vi "smart_home (1).vi"() -> ()   [LabVIEW 2017]
uses:
  <vilib>/MakerHub/LINX/Public/Peripherals/Analog/Analog Read 1 Chan.vi
  <vilib>/MakerHub/LINX/Public/Peripherals/Digital/Digital Write 1 Chan.vi
  <vilib>/MakerHub/LINX/Public/Peripherals/Digital/Digital Read 1 Chan.vi
  <vilib>/MakerHub/LINX/Public/Peripherals/Analog/Analog Read N Chans.vi
  <vilib>/MakerHub/LINX/Public/Peripherals/Digital/Digital Write N Chans.vi
  <vilib>/MakerHub/LINX/Public/Peripherals/Digital/Digital Read N Chans.vi
  <vilib>/MakerHub/LINX/Private/Local IO/LinxAnalogRead.vi
  <vilib>/MakerHub/LINX/Public/Utilities/Check Channel.vi
  <vilib>/MakerHub/LINX/Private/Local IO/LinxDigitalWrite.vi
  <vilib>/MakerHub/LINX/Private/Local IO/LinxDigitalRead.vi
  <vilib>/MakerHub/LINX/Public/Utilities/Open Serial.vi
  <vilib>/MakerHub/LINX/Public/Sensors/Motion/Servo/Servo Open One Channel.vi
  <vilib>/MakerHub/LINX/Public/Sensors/Motion/Servo/Servo Set Pulse Width One Channel.vi
  <vilib>/MakerHub/LINX/Private/Utilties/Generate Error.vi
  <vilib>/MakerHub/LINX/Public/Sensors/Motion/Servo/Servo Close One Channel.vi
  <vilib>/MakerHub/LINX/LMH-LINX.lvlib
  <vilib>/MakerHub/LINX/Public/Sensors/Motion/Servo/Servo.lvlib
panel:
  out "W 5":bool
  out "W 4":bool
  out "W 3":bool
  out "W 2":bool
  out "W 1":bool
  out "Rs/Ro(MQ2)":dbl
  out "Rs(MQ2)":dbl
  out "Boolean":bool
  out "Smoke  Graph":dbl[](graph)
  out "Smoke PPM2":dbl[](array[numeric])
  out "Smoke":dbl(knob) scale=0.0..10000.0
  out "alarm 2":bool
  in  "Servo Channel":u8
  in  "Dial":dbl(knob) scale=500.0..2500.0
  out "Waveform Chart 2":dbl(graph)
  out "Thermometer 2":dbl(slide) scale=0.0..60.0
  in  "Serial Port 2":refnum<visa-resource-name>="N/A"
  in  "Stop Button 2":bool
  in  "LED Value":bool
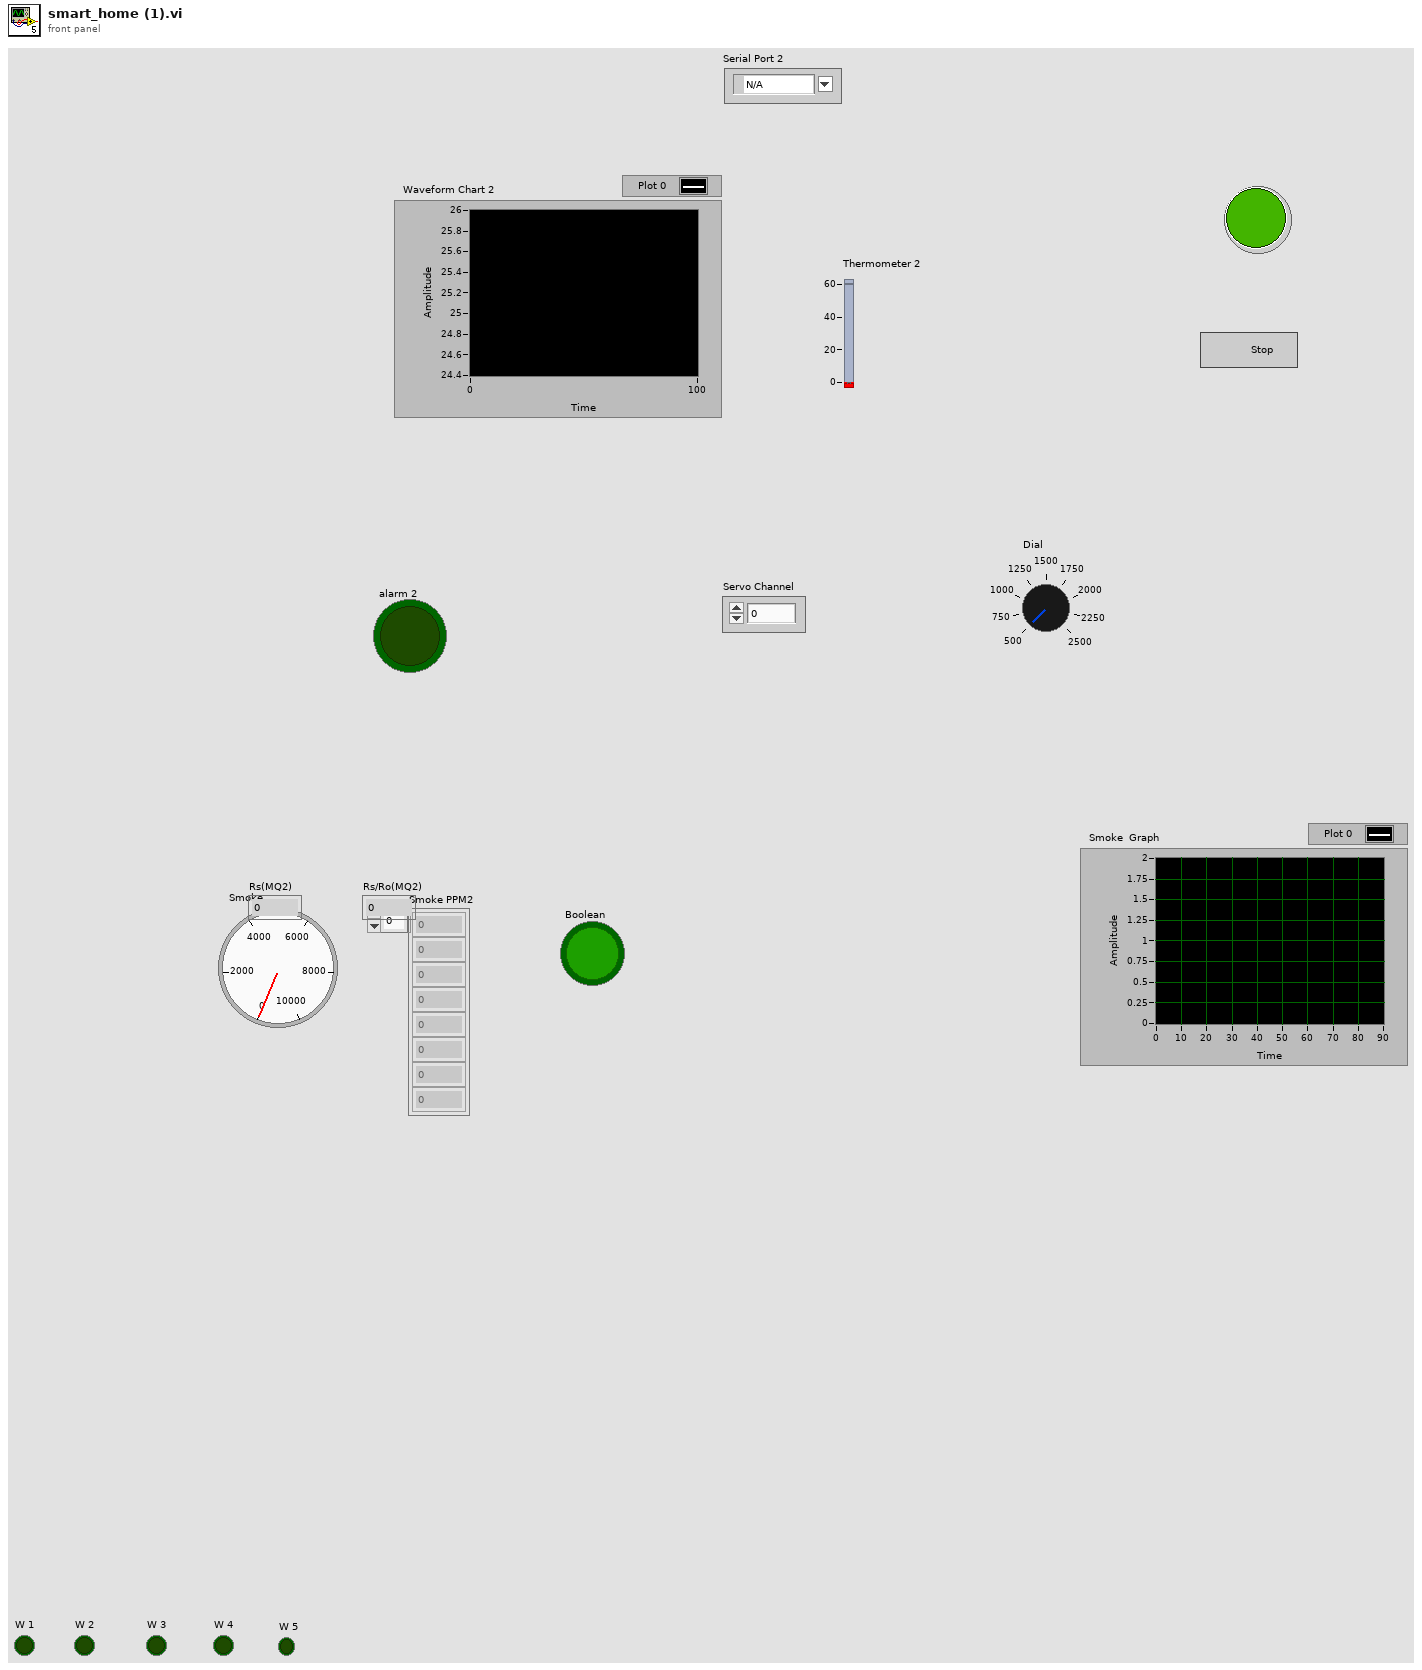
[diagram p1: front panel]
types:
  T1 = typedef "LMH-LINX.lvlib/LINX Ref.ctl" = cluster{"IO":T2, "Interface":T3, "LINX Device Config":T4}
  T2 = typedef "LMH-LINX.lvlib/Platform.ctl" = enum16{"Remote", "Local"}
  T3 = typedef "LMH-LINX.lvlib/Interface.ctl" = enum16{"Serial", "TCP"}
  T4 = typedef "LMH-LINX.lvlib/Device.lvlib/LINX Device Config.ctl" = cluster{"Interface":T3, "COM Port":refnum<visa-resource-name>, "TCP Configuration":T5, "Device Family":u8, "Device ID":u8, "Device Name":string, "TCP Ref":refnum<k5>, "Channels":T6}
  T5 = typedef "LMH-LINX.lvlib/Device.lvlib/TCP Config.ctl" = cluster{"IP Address":string, "Port":u16}
  T6 = typedef "LMH-LINX.lvlib/Channels.ctl" = cluster{"DI":u8[], "DO":u8[], "AI":u8[], "AO":u8[], "PWM":u8[], "QE":u8[], "UART":u8[], "I2C 2":u8[], "SPI":u8[], "CAN":u8[], "Servo":u8[], "AI Ref (V)":dbl, "AI Resolution (Bits)":u8, "AO Ref (V)":dbl, "AO Resolution (Bits)":u8}
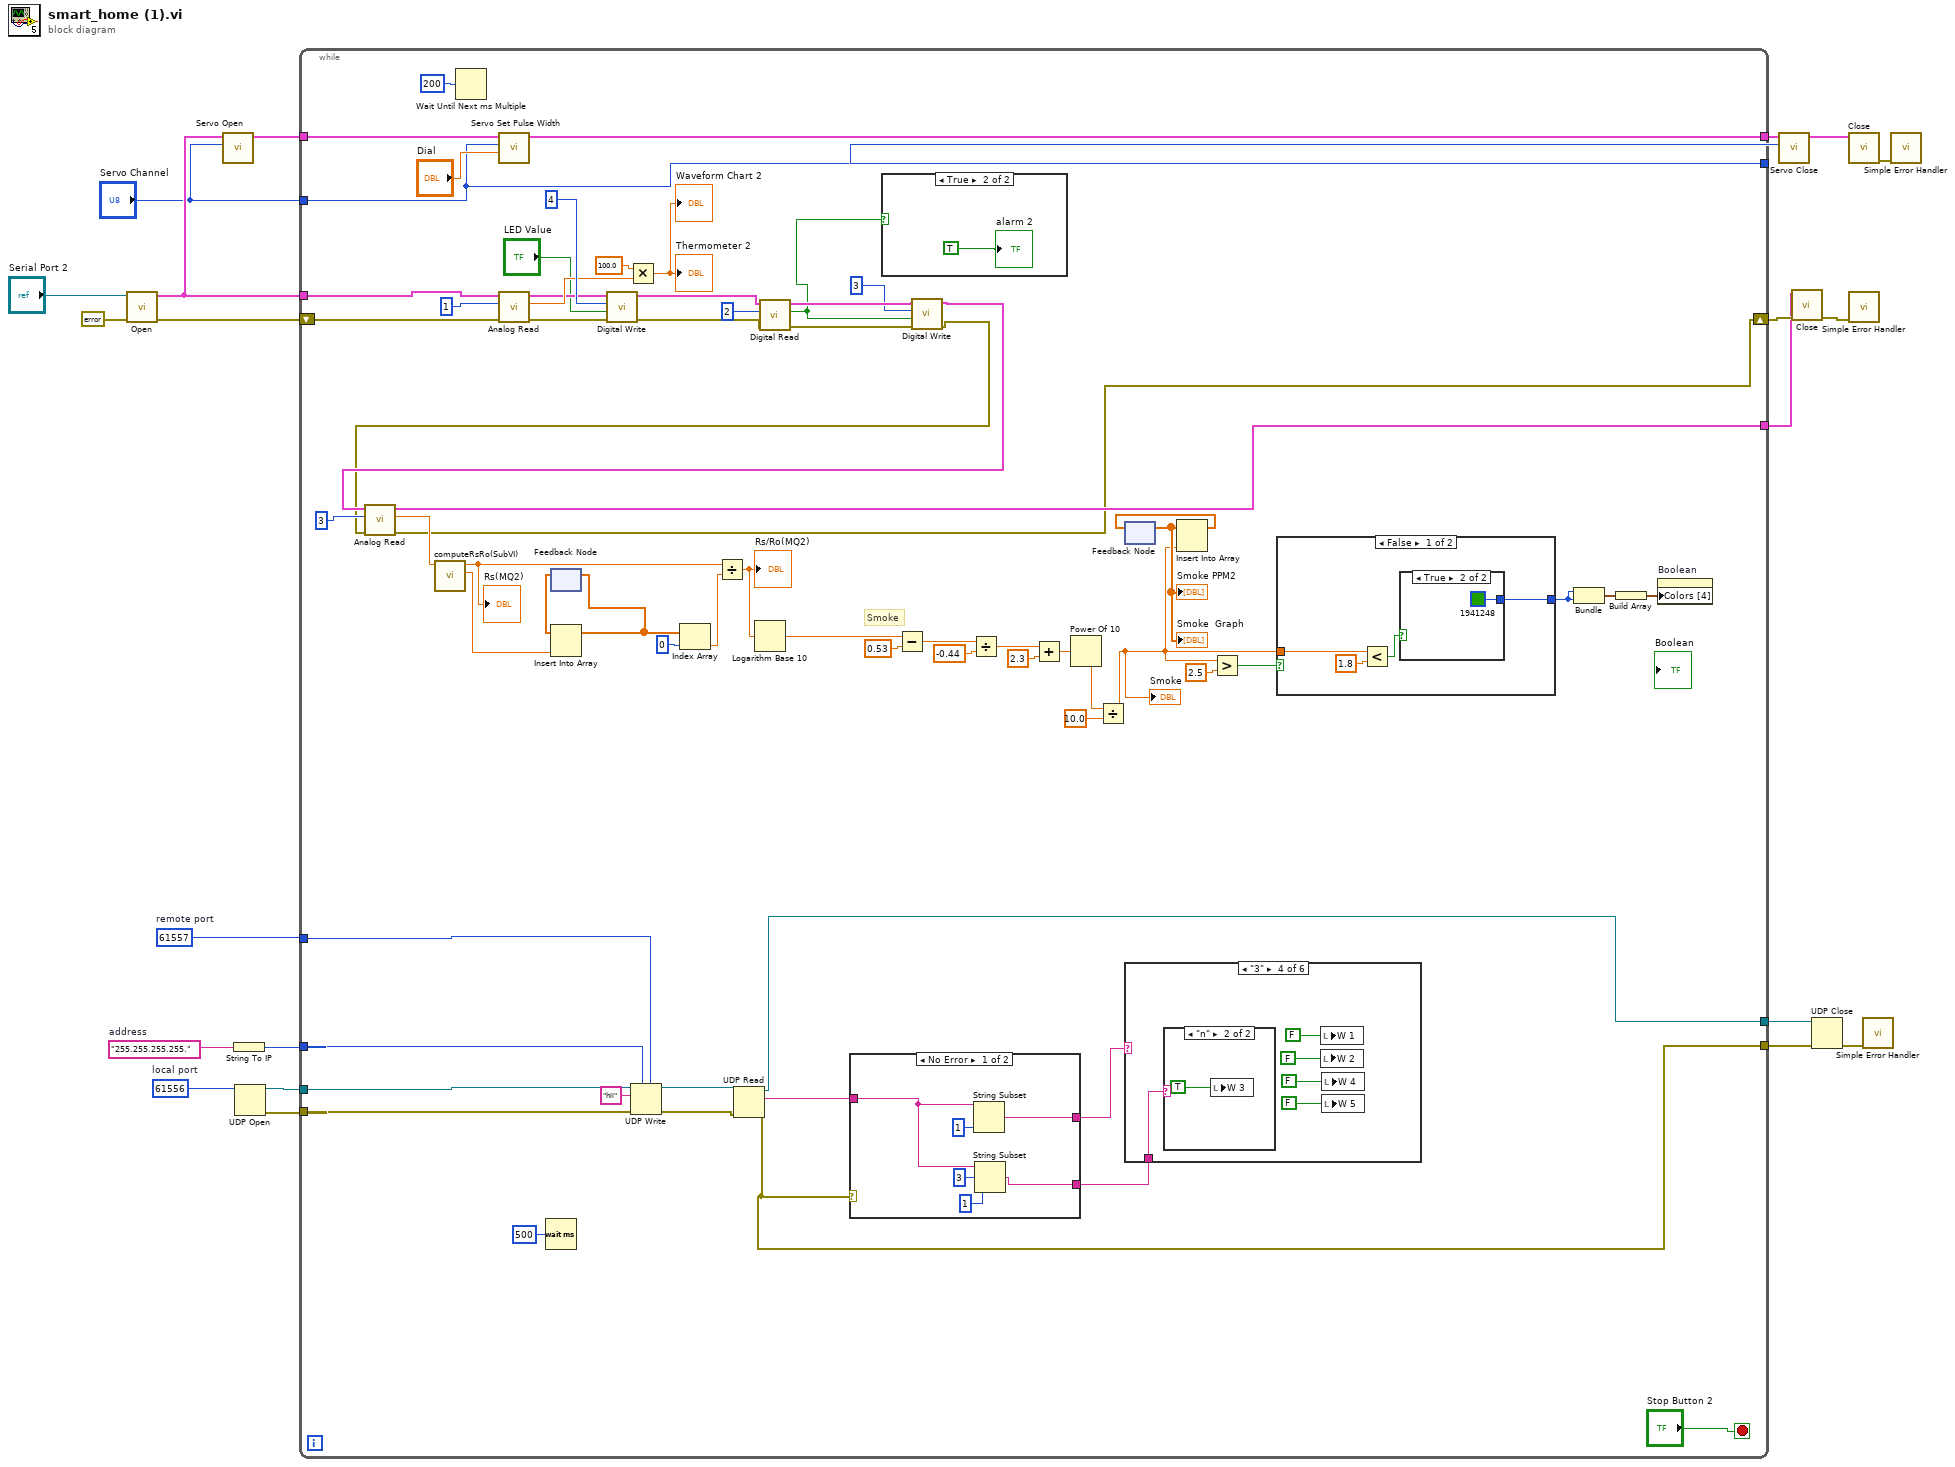
[diagram p0: block diagram]
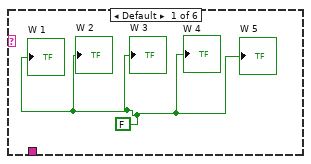
[diagram p2: hidden frame]
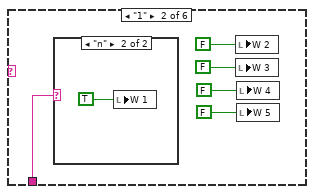
[diagram p3: hidden frame]
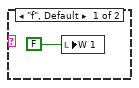
[diagram p4: hidden frame]
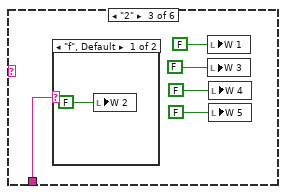
[diagram p5: hidden frame]
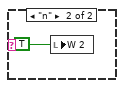
[diagram p6: hidden frame]
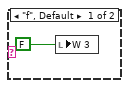
[diagram p7: hidden frame]
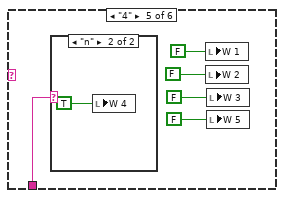
[diagram p8: hidden frame]
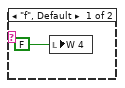
[diagram p9: hidden frame]
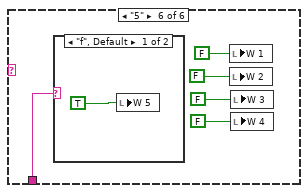
[diagram p10: hidden frame]
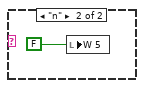
[diagram p11: hidden frame]
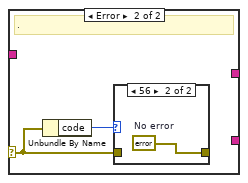
[diagram p12: hidden frame]
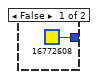
[diagram p14: hidden frame]
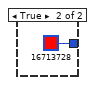
[diagram p15: hidden frame]
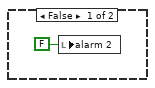
[diagram p16: hidden frame]
diagram:
  w7 = u16 61557  # remote port
  w8 = u16 61556  # local port
  w9 = "255.255.255.255."  # address
  n1 = call-poly <vilib>:"Open.vi"("Error In"=errorcluster {"status"=FALSE, "code"=0, "source"=""}, "Serial Port"="Serial Port 2") -> ("Error Out"=w22:errorcluster, "LINX Resource"=w18:T1)  [unwired: 7 in, 1 out]
  n2 = call-poly <vilib>:"Servo Open.vi"("Servo Channel"="Servo Channel", "LINX Resource"=w18) -> ("LINX Resource"=w17:T1)  [unwired: 8 in, 1 out]
  n3 = String To IP(1:w9) -> (0:w6:u32)
  n4 = UDP Open(11:w8) -> (port=w5:refnum<k16>, 0:w4:errorcluster)  [unwired: 4 in, 1 out]
  n5 = while {
    tunnel: w18 -> [w82]
    shift-right: [w39] -> w21
    shift-left: w22 -> [w80]
    tunnel: w17 -> [w76]
    tunnel: [w75] -> w16
    tunnel: "Servo Channel" -> [w74]
    tunnel: [w74] -> w14
    tunnel: [w41] -> w11
    tunnel: w7 -> [w28]
    tunnel: w6 -> [w27]
    tunnel: w5 -> [w26]
    tunnel: w4 -> [w25]
    tunnel: [w24] -> w2
    tunnel: [w23] -> w1
    stop <- "Stop Button 2" stop-if-true
    # "Smoke"
    n6 = Wait Until Next ms Multiple(millisecond multiple=u32 200) -> ()  [unwired: 1 out]
    n7 = call-poly <vilib>:"Servo Set Pulse Width.vi"("Pulse Width (uS)"="Dial", "Servo Channel"=w74, "LINX Resource"=w76) -> ("LINX Resource"=w75:T1)  [unwired: 7 in, 1 out]
    n8 = call-poly <vilib>:"Analog Read.vi"("Error In"=w80, "Analog Channel"=u8 1 ("DI Channel"), "LINX Resource"=w82) -> ("Error Out"=w79:errorcluster, "Voltage"=w84:dbl, "LINX Resource"=w81:T1)  [unwired: 5 in, 1 out]
    n9 = Wait (ms)(milliseconds to wait=u32 500) -> ()  [unwired: 1 out]
    n10 = feedback #1() -> (w47:dbl[])  [unwired: 1 in]
    n11 = call-poly <vilib>:"Digital Write.vi"("Error In"=w79, "Output Value"="LED Value", "DO Channel"=u8 4 ("Digital Output Channel"), "LINX Resource"=w81) -> ("Error Out"=w72:errorcluster, "LINX Resource"=w73:T1)  [unwired: 6 in]
    n12 = Multiply(x=100.0, y=w84) -> (x*y=→"Thermometer 2" →"Waveform Chart 2":dbl)
    n13 = UDP Write(address=w27, port or service name=w28, connection ID=w26, data in="hii", 8:w25) -> (error out=w32:errorcluster, 3:w33:refnum<k16>)  [unwired: 1 in]
    n14 = UDP Read(connection ID=w33, 8:w32) -> (data out=w29:string, error out=w23:errorcluster, 3:w24:refnum<k16>)  [unwired: 2 in, 2 out]
    n15 = call-poly <vilib>:"Digital Read.vi"("Error In"=w72, "DI Channel"=u8 2, "LINX Resource"=w73) -> ("Error Out"=w69:errorcluster, "DI Value"=w68:bool, "LINX Resource"=w70:T1)  [unwired: 6 in]
    n16 = case shown="No Error" w23 {
      selector: w23 -> [_ w131]
      tunnel: [w127 _] -> w31
      tunnel: [w126 _] -> w30
      tunnel: w29 -> [w125 _]
      frame No Error {
        n17 = String Subset(string=w125, length (rest)=1 ("length (rest)")) -> (substring=w127:string)  [unwired: 1 in]
        n18 = String Subset(string=w125, offset (0)=3, length (rest)=1 ("length (rest)")) -> (substring=w126:string)
      }
      frame Error {
        # "."
        n19 = Unbundle By Name(w131) -> ("code"=w132:i32)
        n20 = case shown="56" w132 {
          tunnel: w131 -> [w133 _]
          tunnel: [w133 w134] -> _
          frame Default {
          }
          frame 56 {
            w134 = errorcluster {"status"=FALSE, "code"=0, "source"=""}  # No error
          }
        }
      }
    }
    n21 = case shown="True" w68 {
      frame False {
        n22 = local write "alarm 2"(FALSE ("alarm 2")) -> ()
      }
      frame True {
        "alarm 2" <- TRUE ("alarm")
      }
    }
    n23 = call-poly <vilib>:"Digital Write.vi"("Error In"=w69, "Output Value"=w68, "DO Channel"=u8 3, "LINX Resource"=w70) -> ("Error Out"=w40:errorcluster, "LINX Resource"=w42:T1)  [unwired: 6 in]
    n24 = call-poly <vilib>:"Analog Read.vi"("Error In"=w40, "Analog Channel"=u8 3, "LINX Resource"=w42) -> ("Error Out"=w39:errorcluster, "Voltage"=w57:dbl, "LINX Resource"=w41:T1)  [unwired: 5 in, 1 out]
    n25 = call "computeRsRo(SubVI).vi"("Voltage"=w57) -> ("Ro"=w48:dbl, "Rs"=w44:dbl)  [unwired: 9 in]
    "Rs(MQ2)" <- w44
    n26 = Insert Into Array "Insert Into Array"(array=w47, new element=w48) -> (w46:dbl[])  [unwired: 1 in]
    n27 = feedback-in #1(w46) -> ()
    n28 = Index Array(array=w46, index=0) -> (element=w45:dbl)
    n29 = Divide(x=w44, y=w45) -> (x/y=w56:dbl)
    "Rs/Ro(MQ2)" <- w56
    n30 = Logarithm Base 10(1:w56) -> (0:w55:dbl)
    n31 = Subtract(x=w55, y=0.53) -> (x-y=w53:dbl)
    n32 = Divide(x=w53, y=-0.44) -> (x/y=w51:dbl)
    n33 = Add(x=w51, y=2.3) -> (x+y=w65:dbl)
    n34 = Power Of 10(x=w65) -> (10^x=w37:dbl)
    n35 = Divide(x=w37, y=10.0) -> (x/y=w38:dbl)
    "Smoke" <- w38
    n36 = feedback #2() -> (w58:dbl[])  [unwired: 1 in]
    "Smoke PPM2" <- w58
    "Smoke  Graph" <- w58
    n37 = case shown="\"3\"" w31 {
      tunnel: w30 -> [_ w90 w97 w104 w111 w118]
      frame Default {
        w89 = FALSE
        "W 5" <- w89
        "W 4" <- w89
        "W 3" <- w89
        "W 2" <- w89
        "W 1" <- w89
      }
      frame "1" {
        n38 = case shown="\"n\"" w90 {
          frame "f", Default {
            n39 = local write "W 1"(FALSE ("Boolean")) -> ()
          }
          frame "n" {
            n40 = local write "W 1"(TRUE ("Boolean")) -> ()
          }
        }
        n41 = local write "W 2"(FALSE ("Boolean 2")) -> ()
        n42 = local write "W 3"(FALSE ("Boolean 3")) -> ()
        n43 = local write "W 4"(FALSE ("Boolean 4")) -> ()
        n44 = local write "W 5"(FALSE ("Boolean 5")) -> ()
      }
      frame "2" {
        n45 = case shown="\"f\", Default" w97 {
          frame "f", Default {
            n46 = local write "W 2"(FALSE ("Boolean 2")) -> ()
          }
          frame "n" {
            n47 = local write "W 2"(TRUE ("Boolean 2")) -> ()
          }
        }
        n48 = local write "W 1"(FALSE ("Boolean")) -> ()
        n49 = local write "W 3"(FALSE ("Boolean 3")) -> ()
        n50 = local write "W 4"(FALSE ("Boolean 4")) -> ()
        n51 = local write "W 5"(FALSE ("Boolean 5")) -> ()
      }
      frame "3" {
        n52 = case shown="\"n\"" w104 {
          frame "f", Default {
            n53 = local write "W 3"(FALSE ("Boolean 3")) -> ()
          }
          frame "n" {
            n54 = local write "W 3"(TRUE ("Boolean 3")) -> ()
          }
        }
        n55 = local write "W 1"(FALSE ("Boolean")) -> ()
        n56 = local write "W 2"(FALSE ("Boolean 2")) -> ()
        n57 = local write "W 4"(FALSE ("Boolean 4")) -> ()
        n58 = local write "W 5"(FALSE ("Boolean 5")) -> ()
      }
      frame "4" {
        n59 = case shown="\"n\"" w111 {
          frame "f", Default {
            n60 = local write "W 4"(FALSE ("Boolean 4")) -> ()
          }
          frame "n" {
            n61 = local write "W 4"(TRUE ("Boolean 4")) -> ()
          }
        }
        n62 = local write "W 1"(FALSE ("Boolean")) -> ()
        n63 = local write "W 2"(FALSE ("Boolean 2")) -> ()
        n64 = local write "W 3"(FALSE ("Boolean 3")) -> ()
        n65 = local write "W 5"(FALSE ("Boolean 5")) -> ()
      }
      frame "5" {
        n66 = case shown="\"f\", Default" w118 {
          frame "f", Default {
            n67 = local write "W 5"(TRUE ("Boolean 6")) -> ()
          }
          frame "n" {
            n68 = local write "W 5"(FALSE ("Boolean 5")) -> ()
          }
        }
        n69 = local write "W 1"(FALSE ("Boolean")) -> ()
        n70 = local write "W 2"(FALSE ("Boolean 2")) -> ()
        n71 = local write "W 3"(FALSE ("Boolean 3")) -> ()
        n72 = local write "W 4"(FALSE ("Boolean 4")) -> ()
      }
    }
    n73 = Insert Into Array(array=w58, new element=w38) -> (w64:dbl[])  [unwired: 1 in]
    n74 = feedback-in #2(w64) -> ()
    n75 = Greater?(x=w38, y=2.5) -> (0:w63:bool)
    n76 = case shown="False" w63 {
      tunnel: [w136 u32 16713728] -> w61
      tunnel: w38 -> [w135 _]
      frame False {
        n77 = Less?(x=w135, y=1.8) -> (x < y?=w138:bool)
        n78 = case shown="True" w138 {
          tunnel: [u32 16772608 u32 1941248] -> w136
          frame False {
          }
          frame True {
          }
        }
      }
      frame True {
      }
    }
    n79 = Bundle(w61, w61) -> (w60:cluster{u32, u32})  [unwired: 1 in]
    n80 = Build Array(w60) -> (w59:cluster{u32, u32}[])
    n81 = property on="Boolean" class="Bool (strict)"("Colors [4]"=w59) -> ()  [unwired: 2 in, 2 out]
  }
  n82 = call-poly <vilib>:"Servo Close.vi"("Servo Channel"=w14, "LINX Resource"=w16) -> ("LINX Resource"=w12:T1)  [unwired: 8 in, 1 out]
  n83 = call <vilib>:"Close.vi"("Error In"=w21, "LINX Resource"=w11) -> ("Error Out"=w20:errorcluster)  [unwired: 9 in]
  n84 = UDP Close(connection ID=w2, 8:w1) -> (error out=w3:errorcluster)  [unwired: 1 out]
  n85 = call <vilib>:"Close.vi"("LINX Resource"=w12) -> ("Error Out"=w13:errorcluster)  [unwired: 10 in]
  n86 = call <vilib>:"Simple Error Handler.vi"("error in (no error)"=w20) -> ()  [unwired: 4 in, 5 out]
  n87 = call <vilib>:"Simple Error Handler.vi"("error in (no error)"=w3) -> ()  [unwired: 4 in, 5 out]
  n88 = call <vilib>:"Simple Error Handler.vi"("error in (no error)"=w13) -> ()  [unwired: 4 in, 5 out]
